vi "initializer_init_controls.vi"(0 "LUA Simulation File":refnum<vi>, 1 "Button Cluster":refnum<vi>, 4 "Cancelled?":refnum<vi>, 5 "Load Button Cluster":refnum<vi>, 8 "LUA Specification File":refnum<vi>, 10 "LUA Validation File":refnum<vi>) -> ()   [LabVIEW 2019]
panel:
  # "*******************************************************************\nBiogas Plant Control\n\nAuthor: Paul Zügel\nGCSC-Frankfurt am Main 2020\n\n*******************************************************************"
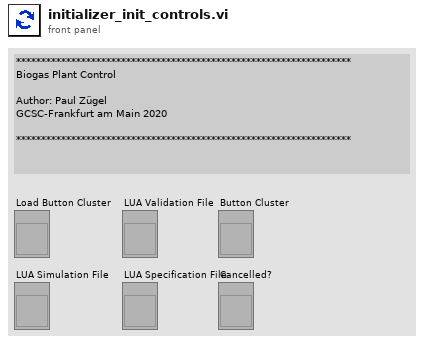
[diagram p1: front panel]
types:
  T1 = enum8{"Enabled", "Disabled", "Disabled and Grayed Out"}
  T2 = cluster{"Save Specs Button":refnum<vi>, "Cancel Button":refnum<vi>, "Run Button":refnum<vi>, "Refresh Button":refnum<vi>, "Validate Button":refnum<vi>}
  T3 = cluster{"Load Vali File":refnum<vi>, "Load Spec File":refnum<vi>, "Load Simulation File":refnum<vi>}
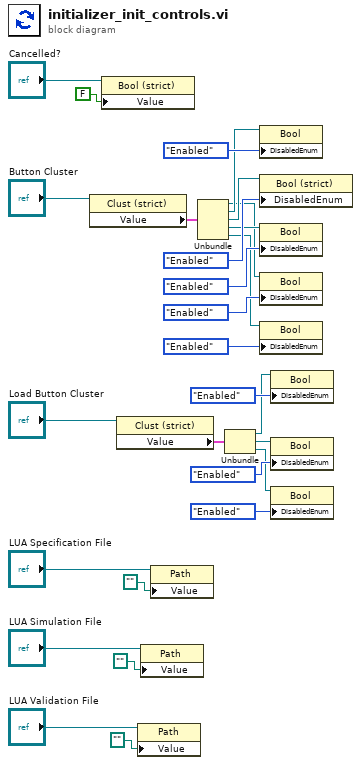
[diagram p0: block diagram]
diagram:
  n1 = property class="Clust (strict)"(reference="Button Cluster") -> ("Value"=w6:T2)  [unwired: 1 in, 2 out]
  n2 = property on="Property Node" class="Bool (strict)"(reference="Cancelled?", "Value"=FALSE ("Stop Button")) -> ()  [unwired: 1 in, 2 out]
  n3 = property class="Clust (strict)"(reference="Load Button Cluster") -> ("Value"=w11:T3)  [unwired: 1 in, 2 out]
  n4 = property class="Path"(reference="LUA Validation File", "Value"=path "") -> ()  [unwired: 1 in, 2 out]
  n5 = property class="Path"(reference="LUA Simulation File", "Value"=path "") -> ()  [unwired: 1 in, 2 out]
  n6 = property class="Path"(reference="LUA Specification File", "Value"=path "") -> ()  [unwired: 1 in, 2 out]
  n7 = Unbundle(w6) -> ("Save Specs Button"=w1:refnum<vi>, "Cancel Button"=w2:refnum<vi>, "Run Button"=w3:refnum<vi>, "Refresh Button"=w5:refnum<vi>, "Validate Button"=w4:refnum<vi>)
  n8 = Unbundle(w11) -> ("Load Vali File"=w10:refnum<vi>, "Load Spec File"=w9:refnum<vi>, "Load Simulation File"=w8:refnum<vi>)
  n9 = property on="Property Node" class="Bool"(reference=w2, "DisabledEnum"=T1."Enabled" ("Disabled")) -> ()  [unwired: 1 in, 2 out]
  n10 = property on="Property Node" class="Bool (strict)"(reference=w3, "DisabledEnum"=T1."Enabled" ("Disabled")) -> ()  [unwired: 1 in, 2 out]
  n11 = property on="Property Node" class="Bool"(reference=w5, "DisabledEnum"=T1."Enabled" ("Disabled")) -> ()  [unwired: 1 in, 2 out]
  n12 = property on="Property Node" class="Bool"(reference=w1, "DisabledEnum"=T1."Enabled" ("Disabled")) -> ()  [unwired: 1 in, 2 out]
  n13 = property on="Property Node" class="Bool"(reference=w4, "DisabledEnum"=T1."Enabled" ("Disabled")) -> ()  [unwired: 1 in, 2 out]
  n14 = property on="Property Node" class="Bool"(reference=w10, "DisabledEnum"=T1."Enabled" ("Disabled")) -> ()  [unwired: 1 in, 2 out]
  n15 = property on="Property Node" class="Bool"(reference=w9, "DisabledEnum"=T1."Enabled" ("Disabled")) -> ()  [unwired: 1 in, 2 out]
  n16 = property on="Property Node" class="Bool"(reference=w8, "DisabledEnum"=T1."Enabled" ("Disabled")) -> ()  [unwired: 1 in, 2 out]
